vi "Spark Manual Control.vi"() -> ()   [LabVIEW 2012]
uses:
  Type/_LC Command.ctl
  <vilib>/Utility/config.llb/Read Key (I32).vi
  <vilib>/Utility/config.llb/Read Key (String).vi
  <vilib>/Utility/config.llb/Read Key (Double).vi
  Server/_Server Global.vi
  Configuration/_Global Configuration.vi
  <vilib>/Utility/config.llb/Write Key (U32).vi
  <vilib>/Utility/config.llb/Write Key (String).vi
  <vilib>/Utility/config.llb/Write Key (Double).vi
  <vilib>/Utility/config.llb/NI_LVConfig.lvlib
panel:
  in  "OvenOff":bool
  in  "OvenOn":bool
  in  "StopPumps":bool
  in  "StartPumps":bool
  in  "Plate\nNumber":u16=1 min=1 max=2 step=1
  out "Spark LC Method File":string
  in  "Inject":bool
  in  "LC-MS Sync":bool=TRUE
  in  "Load":bool
  in  "Injections\n/ Vial":u16=1 min=1 max=100 step=1
  in  "PrepareRun":bool
  in  "Injection\nVolume (uL)":dbl=10.0 min=0.1 max=10000.0 step=1.0
  in  "Vial\nNumber":string="A1"
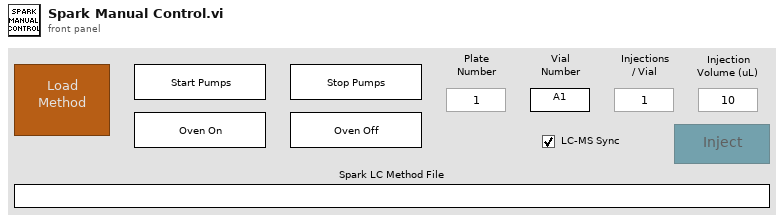
[diagram p1: front panel]
types:
  T1 = enum8{"Enabled", "Disabled", "Disabled and Grayed Out"}
  T2 = enum32{"existing file", "new file", "new or existing file", "existing dir", "new dir", "new or existing dir", "existing file (use LLBs)", "new file (use LLBs)", "new or existing file (use LLBs)", "new or existing file or directory (use LLBs)"}
  T3 = typedef "_LC Command.ctl" = enum16{"No Command", "Initialize", "Get Configuration", "Get Status", "Get LC Method Contents", "Oven OnOff", "Pump OnOFF", "Rinse Autosampler", "Run Sample", "Set EnvParameters", "Set Method", "Start Equilibration", "Stop Run", "Get LastError", "Clear Error", "Close"}
  T4 = typedef "NI_LVConfig.lvlib/Config Data RefNum.ctl" = refnum<k1>
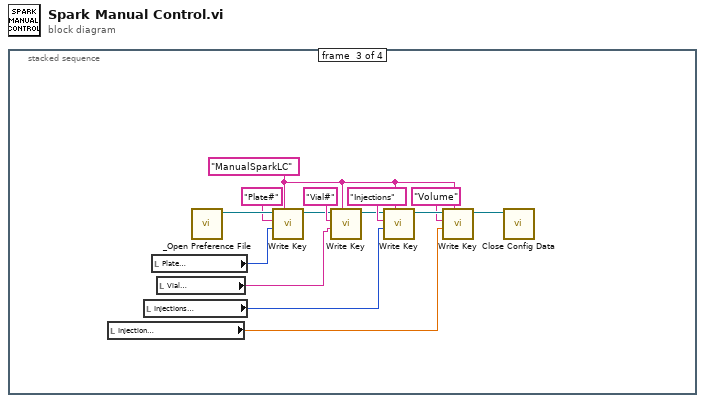
[diagram p0: block diagram]
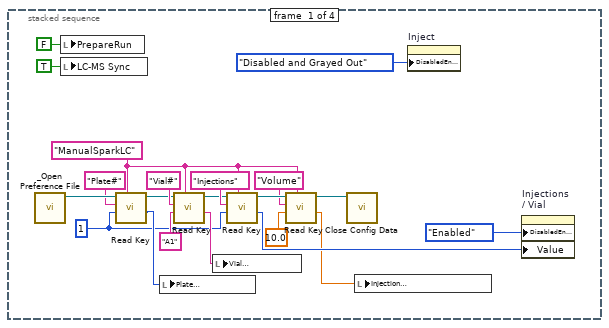
[diagram p2: hidden frame]
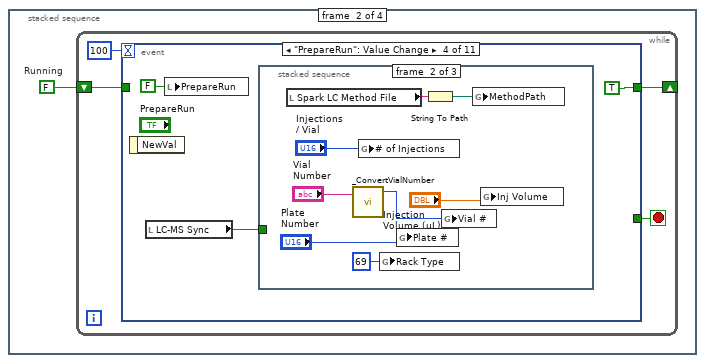
[diagram p3: hidden frame]
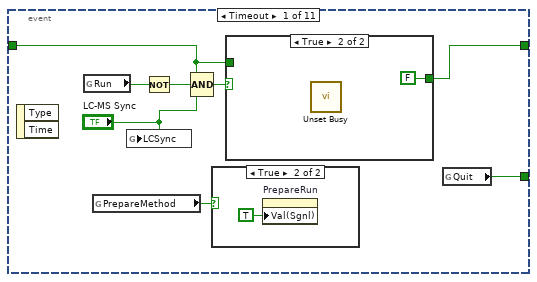
[diagram p4: hidden frame]
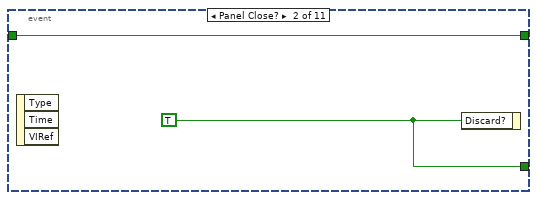
[diagram p7: hidden frame]
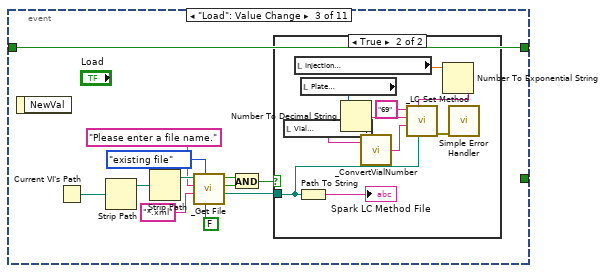
[diagram p8: hidden frame]
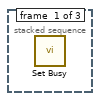
[diagram p10: hidden frame]
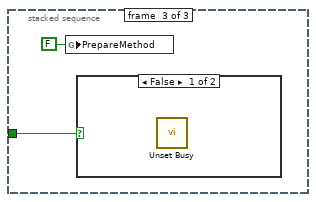
[diagram p11: hidden frame]
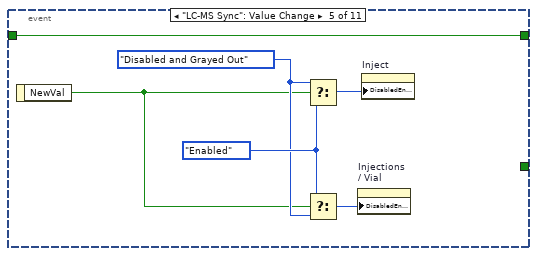
[diagram p13: hidden frame]
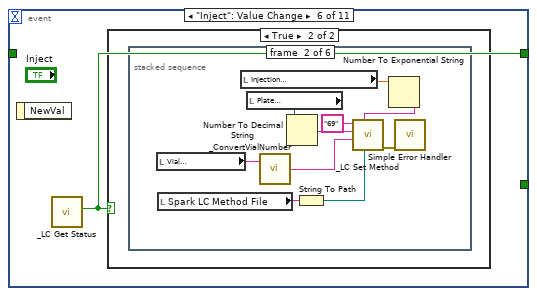
[diagram p14: hidden frame]
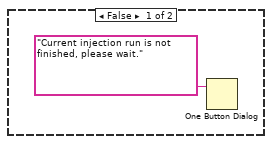
[diagram p15: hidden frame]
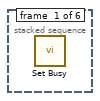
[diagram p16: hidden frame]
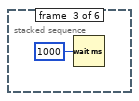
[diagram p17: hidden frame]
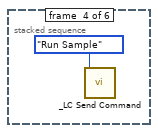
[diagram p18: hidden frame]
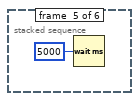
[diagram p19: hidden frame]
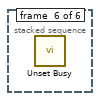
[diagram p20: hidden frame]
diagram:
  n1 = stacked-sequence {
    frame #0 {
      w4 = 1 ("Plate\nNumber")
      w15 = "ManualSparkLC" ("section")
      n2 = call "_Open Preference File.vi"() -> ("refnum"=w10:T4)  [unwired: 1 in, 6 out]
      n3 = local write "PrepareRun"(FALSE ("PrepareRun")) -> ()
      n4 = local write "LC-MS Sync"(TRUE ("LC-MS Sync")) -> ()
      n5 = call-poly <vilib>:"Read Key.vi"("section"=w15, "default value"=w4, "key"="Plate#" ("section"), "refnum"=w10) -> ("value"=w6:i32, "refnum out"=w9:T4)  [unwired: 4 in, 2 out]
      n6 = local write "Plate\nNumber"(w6) -> ()
      n7 = call-poly <vilib>:"Read Key.vi"("section"=w15, "default value"="A1" ("Vial\nNumber"), "key"="Vial#" ("section"), "refnum"=w9) -> ("value"=w5:string, "refnum out"=w12:T4)  [unwired: 4 in, 2 out]
      n8 = local write "Vial\nNumber"(w5) -> ()
      n9 = call-poly <vilib>:"Read Key.vi"("section"=w15, "default value"=w4, "key"="Injections" ("section"), "refnum"=w12) -> ("value"=w3:i32, "refnum out"=w16:T4)  [unwired: 4 in, 2 out]
      n10 = call-poly <vilib>:"Read Key.vi"("section"=w15, "default value"=10.0 ("Injection\nVolume (uL)"), "key"="Volume" ("section"), "refnum"=w16) -> ("value"=w1:dbl, "refnum out"=w17:T4)  [unwired: 4 in, 2 out]
      n11 = call <vilib>:"Close Config Data.vi"("refnum"=w17) -> ()  [unwired: 2 in, 9 out]
      n12 = local write "Injection\nVolume (uL)"(w1) -> ()
      n13 = property on="Inject" class="Bool"("DisabledEnum"=T1."Disabled and Grayed Out" ("Disabled")) -> ()  [unwired: 2 in, 2 out]
      n14 = property on="Injections\n/ Vial" class="DigNum (strict)"("DisabledEnum"=T1."Enabled" ("Disabled"), "Value"=w3) -> ()  [unwired: 2 in, 2 out]
    }
    frame #1 {
      w22 = FALSE  # Running
      n15 = while {
        shift-right: [w24] -> _
        shift-left: w22 -> [w23]
        stop <- w25 stop-if-true
        n16 = event shown="[3] \"PrepareRun\": Value Change" {
          selector: _ -> [_ _ _ _ _ _ _ _ _ _ _]
          dyn-events: _ -> [_ _ _ _ _ _ _ _ _ _ _]
          timeout: 100 -> [_ _ _ _ _ _ _ _ _ _ _]
          tunnel: [w34 w39 _ _ _ _ _ _ _ _ _] -> w25
          tunnel: [w28 w38 w40 TRUE w80 w81 w96 w102 w107 w112 w117] -> w24
          tunnel: w23 -> [w29 w38 w40 _ w80 _ w96 w102 w107 w112 w117]
          event Timeout {
            n17 = event-data() -> ()  [unwired: 1 in, 2 out]
            n18 = global read "_Global Configuration.vi" "Run"() -> (w32:bool)
            n19 = global read "_Server Global.vi" "PrepareMethod"() -> (w33:bool)
            n20 = global write "_Server Global.vi" "LCSync"("LC-MS Sync") -> ()
            n21 = Not(x=w32) -> (.not. x?=w31:bool)
            n22 = Compound Arithmetic op=AND(w29, w31, "LC-MS Sync") -> (w30:bool)
            n23 = case shown="True" w33 {
              frame False {
              }
              frame True {
                n24 = property on="PrepareRun" class="Bool (strict)"("Val(Sgnl)"=TRUE ("Value (Signaling)")) -> ()  [unwired: 2 in, 2 out]
              }
            }
            n25 = case shown="True" w30 {
              tunnel: [w35 FALSE] -> w28
              tunnel: w29 -> [w35 _]
              frame False {
              }
              frame True {
                n26 = call <vilib>:"Unset Busy.vi"() -> ()  [unwired: 11 in, 1 out]
              }
            }
            n27 = global read "_Global Configuration.vi" "Quit"() -> (w34:bool)
          }
          event Panel Close? {
            w39 = TRUE ("Discard?")
            n28 = event-data() -> ()  [unwired: 1 in, 3 out]
            n29 = event-data("Discard?"=w39) -> ()  [unwired: 1 in, 1 out]
          }
          event "Load": Value Change {
            n30 = event-data() -> ()  [unwired: 1 in, 1 out]
            n31 = Current VI's Path() -> (path=w51:path)
            n32 = Strip Path(path=w51) -> (stripped path=w50:path)  [unwired: 1 out]
            n33 = Strip Path(path=w50) -> (stripped path=w49:path)  [unwired: 1 out]
            n34 = call "_Get File.vi"("For Write (T)"=FALSE, "select mode (new or existing)"=T2."existing file", "extension (isd)"="*.xml", "prompt"="Please enter a file name.", "Start Path"=w49) -> ("Seleted File"=w46:path, "Exists"=w42:bool, "Succeeded"=w43:bool)  [unwired: 2 in]
            n35 = And(x=w43, y=w42) -> (x .and. y?=w41:bool)
            n36 = case shown="True" w41 {
              tunnel: w46 -> [_ w60]
              frame False {
              }
              frame True {
                n37 = local read "Vial\nNumber"() -> (w52:string)
                n38 = local read "Injection\nVolume (uL)"() -> (w58:dbl)
                n39 = Path To String(path=w60) -> (string=→"Spark LC Method File":string)
                n40 = local read "Plate\nNumber"() -> (w55:u16)
                n41 = Number To Decimal String(number=w55) -> (decimal integer string=w54:string)  [unwired: 1 in]
                n42 = call "_ConvertVialNumber.vi"("Vial#"=w52) -> ("NumericVial# 2"=w53:string)  [unwired: 1 in, 2 out]
                n43 = Number To Exponential String(number=w58) -> (E-format string=w57:string)  [unwired: 3 in]
                n44 = call "_LC Set Method.vi"("Path"=w60, "Injection Volume"=w57, "Vial Number"=w53, "Plate Number"=w54, "Rack Type"="69") -> ("error out"=w59:errorcluster)  [unwired: 2 in, 4 out]
                n45 = call <vilib>:"Simple Error Handler.vi"("error in (no error)"=w59) -> ()  [unwired: 4 in, 5 out]
              }
            }
          }
          event "PrepareRun": Value Change {
            n46 = event-data() -> ()  [unwired: 1 in, 1 out]
            n47 = local read "LC-MS Sync"() -> (w62:bool)
            n48 = local write "PrepareRun"(FALSE ("PrepareRun")) -> ()
            n49 = stacked-sequence {
              tunnel: w62 -> [_ _ w73]
              frame #0 {
                n50 = call <vilib>:"Set Busy.vi"() -> ()  [unwired: 10 in, 2 out]
              }
              frame #1 {
                n51 = local read "Spark LC Method File"() -> (w68:string)
                n52 = call "_ConvertVialNumber.vi"("Vial#"="Vial\nNumber") -> ("NumericVial#"=w65:u16)  [unwired: 1 in, 2 out]
                n53 = global write "_Server Global.vi" "# of Injections"("Injections\n/ Vial") -> ()
                n54 = global write "_Server Global.vi" "Rack Type"(u16 69 ("Rack Type")) -> ()
                n55 = global write "_Server Global.vi" "Plate #"("Plate\nNumber") -> ()
                n56 = String To Path(string=w68) -> (path=w67:path)
                n57 = global write "_Server Global.vi" "Vial #"(w65) -> ()
                n58 = global write "_Server Global.vi" "MethodPath"(w67) -> ()
                n59 = global write "_Server Global.vi" "Inj Volume"("Injection\nVolume (uL)") -> ()
              }
              frame #2 {
                n60 = global write "_Server Global.vi" "PrepareMethod"(FALSE ("PrepareMethod")) -> ()
                n61 = case shown="False" w73 {
                  frame False {
                    n62 = call <vilib>:"Unset Busy.vi"() -> ()  [unwired: 11 in, 1 out]
                  }
                  frame True {
                  }
                }
              }
            }
          }
          event "LC-MS Sync": Value Change {
            w79 = T1."Enabled" ("Disabled")
            w78 = T1."Disabled and Grayed Out" ("Disabled")
            n63 = event-data() -> ("NewVal"=w76:bool)  [unwired: 1 in]
            n64 = Select(t=w78, s=w76, f=w79) -> (s? t:f=w77:T1)
            n65 = Select(t=w79, s=w76, f=w78) -> (s? t:f=w75:T1)
            n66 = property on="Injections\n/ Vial" class="DigNum (strict)"("DisabledEnum"=w75) -> ()  [unwired: 2 in, 2 out]
            n67 = property on="Inject" class="Bool"("DisabledEnum"=w77) -> ()  [unwired: 2 in, 2 out]
          }
          event "Inject": Value Change {
            n68 = event-data() -> ()  [unwired: 1 in, 1 out]
            n69 = call "_LC Get Status.vi"() -> ("Ready"=w81:bool)  [unwired: 4 in, 4 out]
            n70 = case shown="True" w81 {
              frame False {
                n71 = One Button Dialog(message="Current injection run is not finished, please wait.") -> ()  [unwired: 1 in, 1 out]
              }
              frame True {
                n72 = stacked-sequence {
                  frame #0 {
                    n73 = call <vilib>:"Set Busy.vi"() -> ()  [unwired: 10 in, 2 out]
                  }
                  frame #1 {
                    n74 = local read "Vial\nNumber"() -> (w84:string)
                    n75 = local read "Spark LC Method File"() -> (w86:string)
                    n76 = local read "Injection\nVolume (uL)"() -> (w91:dbl)
                    n77 = local read "Plate\nNumber"() -> (w88:u16)
                    n78 = call "_ConvertVialNumber.vi"("Vial#"=w84) -> ("NumericVial# 2"=w83:string)  [unwired: 1 in, 2 out]
                    n79 = Number To Decimal String(number=w88) -> (decimal integer string=w87:string)  [unwired: 1 in]
                    n80 = String To Path(string=w86) -> (path=w85:path)
                    n81 = Number To Exponential String(number=w91) -> (E-format string=w90:string)  [unwired: 3 in]
                    n82 = call "_LC Set Method.vi"("Path"=w85, "Injection Volume"=w90, "Vial Number"=w83, "Plate Number"=w87, "Rack Type"="69") -> ("error out"=w92:errorcluster)  [unwired: 2 in, 4 out]
                    n83 = call <vilib>:"Simple Error Handler.vi"("error in (no error)"=w92) -> ()  [unwired: 4 in, 5 out]
                  }
                  frame #2 {
                    n84 = Wait (ms)(milliseconds to wait=u32 1000) -> ()  [unwired: 1 out]
                  }
                  frame #3 {
                    n85 = call "_LC Send Command.vi"("Command"=_LC_Command."Run Sample") -> ()  [unwired: 9 in, 2 out]
                  }
                  frame #4 {
                    n86 = Wait (ms)(milliseconds to wait=u32 5000) -> ()  [unwired: 1 out]
                  }
                  frame #5 {
                    n87 = call <vilib>:"Unset Busy.vi"() -> ()  [unwired: 11 in, 1 out]
                  }
                }
              }
            }
          }
          event "Vial\nNumber": Value Change {
            n88 = event-data() -> ("NewVal"=w99:string, "OldVal"=w97:string)  [unwired: 1 in]
            n89 = call "_ConvertVialNumber.vi"("Vial#"=w99) -> ("Valid"=w98:bool)  [unwired: 1 in, 2 out]
            n90 = case shown="False" w98 {
              tunnel: w97 -> [w101 _]
              frame False {
                n91 = local write "Vial\nNumber"(w101) -> ()
                n92 = One Button Dialog(message="Vial Number must be within the range between A1 and P24.") -> ()  [unwired: 1 in, 1 out]
              }
              frame True {
              }
            }
          }
          event "StartPumps": Value Change {
            n93 = event-data() -> ()  [unwired: 1 in, 1 out]
            n94 = case shown="False" w102 {
              frame False {
                n95 = call "_LC Send Command.vi"("Parameter"="1" ("String In"), "Command"=_LC_Command."Pump OnOFF") -> ("error out"=w104:errorcluster)  [unwired: 8 in, 1 out]
                n96 = call <vilib>:"Simple Error Handler.vi"("error in (no error)"=w104) -> ()  [unwired: 1 in, 8 out]
              }
              frame True {
                n97 = One Button Dialog(message="Start Pumps button is disabled during a run.") -> ()  [unwired: 1 in, 1 out]
              }
            }
          }
          event "StopPumps": Value Change {
            n98 = event-data() -> ()  [unwired: 1 in, 1 out]
            n99 = case shown="False" w107 {
              frame False {
                n100 = call "_LC Send Command.vi"("Parameter"="0" ("String In"), "Command"=_LC_Command."Pump OnOFF") -> ("error out"=w109:errorcluster)  [unwired: 8 in, 1 out]
                n101 = call <vilib>:"Simple Error Handler.vi"("error in (no error)"=w109) -> ()  [unwired: 1 in, 8 out]
              }
              frame True {
                n102 = One Button Dialog(message="Stop Pumps button is disabled during a run.") -> ()  [unwired: 1 in, 1 out]
              }
            }
          }
          event "OvenOn": Value Change {
            n103 = event-data() -> ()  [unwired: 1 in, 1 out]
            n104 = case shown="False" w112 {
              frame False {
                n105 = call "_LC Send Command.vi"("Parameter"="1" ("String In"), "Command"=_LC_Command."Oven OnOff") -> ("error out"=w114:errorcluster)  [unwired: 8 in, 1 out]
                n106 = call <vilib>:"Simple Error Handler.vi"("error in (no error)"=w114) -> ()  [unwired: 1 in, 8 out]
              }
              frame True {
                n107 = One Button Dialog(message="Oven On button is disabled during a run.") -> ()  [unwired: 1 in, 1 out]
              }
            }
          }
          event "OvenOff": Value Change {
            n108 = event-data() -> ()  [unwired: 1 in, 1 out]
            n109 = case shown="False" w117 {
              frame False {
                n110 = call "_LC Send Command.vi"("Parameter"="0" ("String In"), "Command"=_LC_Command."Oven OnOff") -> ("error out"=w119:errorcluster)  [unwired: 8 in, 1 out]
                n111 = call <vilib>:"Simple Error Handler.vi"("error in (no error)"=w119) -> ()  [unwired: 1 in, 8 out]
              }
              frame True {
                n112 = One Button Dialog(message="Oven Off button is disabled during a run.") -> ()  [unwired: 1 in, 1 out]
              }
            }
          }
        }
      }
    }
    frame #2 {
      w133 = "ManualSparkLC" ("section")
      n113 = local read "Injection\nVolume (uL)"() -> (w122:dbl)
      n114 = local read "Injections\n/ Vial"() -> (w123:u16)
      n115 = local read "Plate\nNumber"() -> (w125:u16)
      n116 = local read "Vial\nNumber"() -> (w124:string)
      n117 = call "_Open Preference File.vi"() -> ("refnum"=w128:T4)  [unwired: 1 in, 6 out]
      n118 = call-poly <vilib>:"Write Key.vi"("section"=w133, "value"=w125, "key"="Plate#" ("section"), "refnum"=w128) -> ("refnum out"=w127:T4)  [unwired: 5 in, 2 out]
      n119 = call-poly <vilib>:"Write Key.vi"("section"=w133, "value"=w124, "key"="Vial#" ("section"), "refnum"=w127) -> ("refnum out"=w130:T4)  [unwired: 5 in, 2 out]
      n120 = call-poly <vilib>:"Write Key.vi"("section"=w133, "value"=w123, "key"="Injections" ("section"), "refnum"=w130) -> ("refnum out"=w134:T4)  [unwired: 5 in, 2 out]
      n121 = call-poly <vilib>:"Write Key.vi"("section"=w133, "value"=w122, "key"="Volume" ("section"), "refnum"=w134) -> ("refnum out"=w135:T4)  [unwired: 5 in, 2 out]
      n122 = call <vilib>:"Close Config Data.vi"("refnum"=w135) -> ()  [unwired: 2 in, 9 out]
    }
    frame #3 {
      n123 = property class="VI"("Front Panel.Open"=FALSE ("Front Panel Window:Open")) -> ()  [unwired: 2 in, 2 out]
    }
  }
